vi "AFTSChildForm.vi"() -> ()   [LabVIEW 2012]
panel:
  in  "Tab Control":T1(tab)
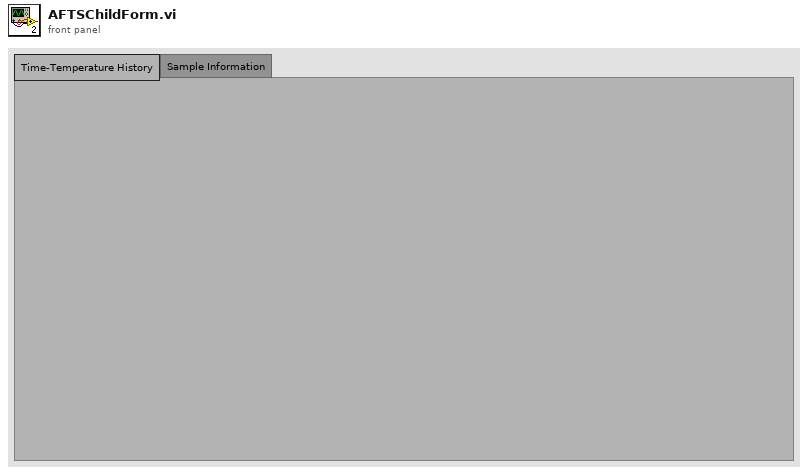
[diagram p1: front panel]
types:
  T1 = enum32{"Time-Temperature History", "Sample Information"}
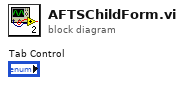
[diagram p0: block diagram]
diagram:
